vi "G.vi"(3 "t":dbl, 4 "n^2":dbl, 5 "Promien krzywizny południka [v]":dbl, 6 "fi[rad]":dbl) -> (0 "G":dbl)   [LabVIEW 2015, in "Biblioteka moduł map v3.lvlib" / "Konwersja wsp.lvlib" / "UTM.lvlib" / "Konwersja na UTM.lvlib"]
doc: "Współczynnik wzoru na konwersję na UTM."
uses:
  Konwersja na UTM.lvlib
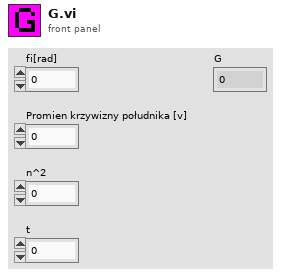
[diagram p1: front panel]
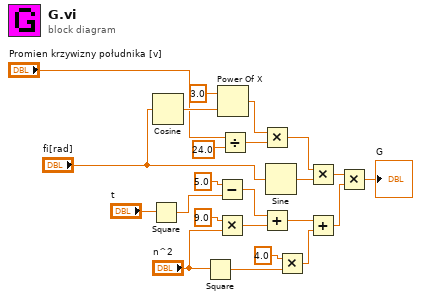
[diagram p0: block diagram]
diagram:
  n1 = Square(x="t") -> (x^2=w13:dbl)
  n2 = Cosine(x="fi[rad]") -> (cos(x)=w19:dbl)
  n3 = Square(x="n^2") -> (x^2=w6:dbl)
  n4 = Subtract(x=5.0, y=w13) -> (x-y=w10:dbl)
  n5 = Multiply(x=9.0, y="n^2") -> (x*y=w9:dbl)
  n6 = Power Of X(1:w19, 2:3.0 ("y")) -> (0:w21:dbl)
  n7 = Divide(x="Promien krzywizny południka [v]", y=24.0) -> (x/y=w22:dbl)
  n8 = Multiply(x=w21, y=w22) -> (x*y=w23:dbl)
  n9 = Add(x=w10, y=w9) -> (x+y=w8:dbl)
  n10 = Sine(x="fi[rad]") -> (sin(x)=w15:dbl)
  n11 = Multiply(x=4.0, y=w6) -> (x*y=w5:dbl)
  n12 = Multiply(x=w23, y=w15) -> (x*y=w2:dbl)
  n13 = Add(x=w8, y=w5) -> (x+y=w3:dbl)
  n14 = Multiply(x=w2, y=w3) -> (x*y=→"G":dbl)
